vi "Main_SubVI_Comment to Hex.vi"(8 "Error In":errorcluster, 11 "Normal In":string) -> (0 "Error Out":errorcluster, 3 "Hex Out":string)   [LabVIEW 2015]
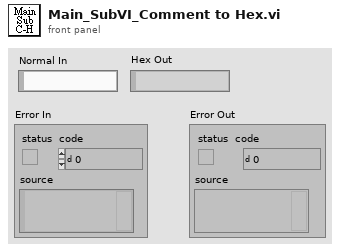
[diagram p1: front panel]
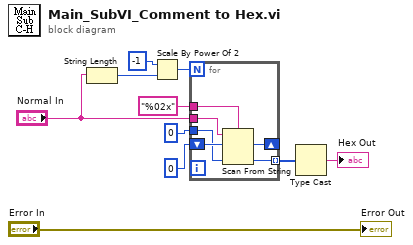
[diagram p0: block diagram]
diagram:
  n1 = String Length(string="Normal In") -> (length=w8:i32)
  n2 = Scale By Power Of 2(n=-1, x=w8) -> (x*2^n=w6:i32)
  n3 = for {
    N: w6 -> [_]
    shift-right: [w15] -> _
    shift-left: u32 0 -> [w16]
    tunnel: "Normal In" -> [w14]
    tunnel: u8 0 ("U8") -> [w13]
    tunnel: [w12] -> w4 mode=indexing
    tunnel: "%02x" ("format string") -> [w11]
    n4 = Scan From String(format string=w11, input string=w14, initial scan location=w16, default 1=w13) -> (offset past scan=w15:u32, output 1=w12:u8)  [unwired: 1 in, 2 out]
  }
  n5 = Type Cast(x=w4) -> (*(type *) &x=→"Hex Out":string)  [unwired: 1 out]
  "Error Out" <- "Error In"
